vi "Read Path.vi"(11 "SolutionBuilder in":refnum<class "SolutionBuilder.lvclass">) -> (2 "Path":path, 3 "SolutionBuilder out":refnum<class "SolutionBuilder.lvclass">)   [LabVIEW 2019, in "SolutionBuilder.lvlib" / "SolutionBuilder.lvclass"]
uses:
  SolutionBuilder.lvclass
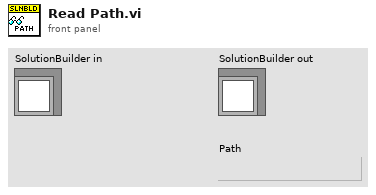
[diagram p1: front panel]
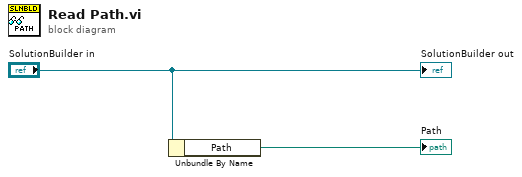
[diagram p0: block diagram]
diagram:
  n1 = Unbundle By Name("SolutionBuilder in") -> ("Path"=→"Path":path)
  "SolutionBuilder out" <- "SolutionBuilder in"
